vi "Check Status.vi"(8 "error in (no error)":errorcluster, 11 "Lockin SR830 in":refnum<class "Lockin SR830.lvclass">) -> (0 "error out":errorcluster, 1 "Status":string, 2 "Ready?":bool, 3 "Lockin SR830 out":refnum<class "Lockin SR830.lvclass">)   [LabVIEW 2015, in "Lockin SR830.lvclass"]
doc: "Checks if the instrument is powered on and updates its member data with the instrument's current status."
uses:
  Lockin SR830.lvclass
  Utility Classes/Readable/Readable.lvclass
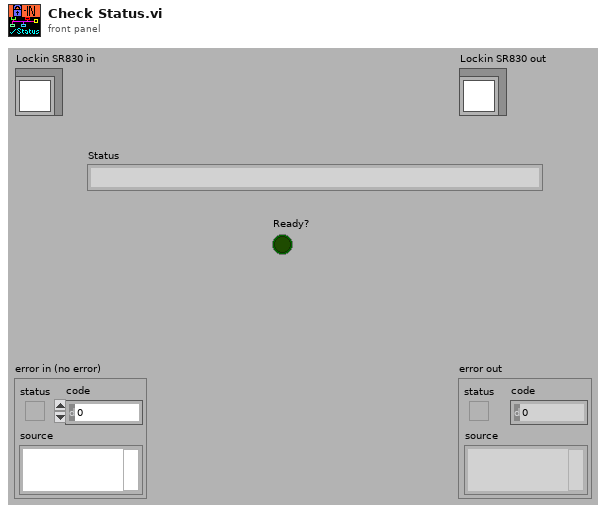
[diagram p1: front panel]
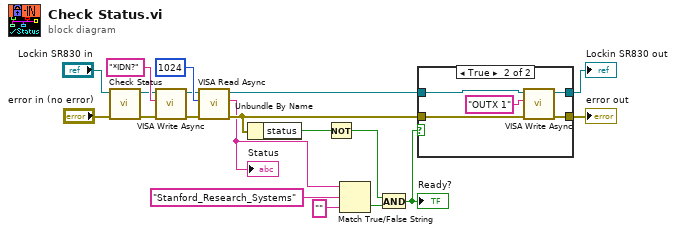
[diagram p0: block diagram]
diagram:
  n1 = call-parent "Check Status.vi"("error in (no error)"="error in (no error)", "Instrument in"="Lockin SR830 in") -> ("error out"=w7:errorcluster, "Instrument out"=w6:refnum<class "Lockin SR830.lvclass">)  [unwired: 8 out]
  n2 = call-dynamic "VISA Write Async.vi"("error in (no error)"=w7, "write buffer"="*IDN?", "Instrument in"=w6) -> ("error out"=w16:errorcluster, "Instrument out"=w8:refnum<class "Lockin SR830.lvclass">)  [unwired: 7 out]
  n3 = call-dynamic "VISA Read Async.vi"("error in (no error)"=w16, "byte count"=1024, "Instrument in"=w8) -> ("error out"=w3:errorcluster, "read buffer"=w1:string, "Instrument out"=w5:refnum<class "Lockin SR830.lvclass">)  [unwired: 6 out]
  "Status" <- w1
  n4 = Unbundle By Name(w3) -> ("status"=w12:bool)
  n5 = Not(x=w12) -> (.not. x?=w10:bool)
  n6 = Match True/False String(2:"", 3:"Stanford_Research_Systems", 4:w1) -> (0:w11:bool)  [unwired: 1 out]
  n7 = And(x=w10, y=w11) -> (x .and. y?=w9:bool)
  "Ready?" <- w9
  n8 = case shown="True" w9 {
    tunnel: w5 -> [w20 w25]
    tunnel: [w20 w24] -> w4
    tunnel: [w21 w23] -> w2
    tunnel: w3 -> [w21 w22]
    frame False {
    }
    frame True {
      n9 = call-dynamic "VISA Write Async.vi"("error in (no error)"=w22, "write buffer"="OUTX 1", "Instrument in"=w25) -> ("error out"=w23:errorcluster, "Instrument out"=w24:refnum<class "Lockin SR830.lvclass">)  [unwired: 7 out]
    }
  }
  "error out" <- w2
  "Lockin SR830 out" <- w4
